vi "Interpolate Tach Pulses.vi"(5 "reset? (True)":bool=TRUE, 6 "avg on n pulses (1:no average)":i32=1, 8 "error in (no error)":errorcluster, 9 "pulse/revolution wanted":dbl=4.0 format="%.2f", 10 "pulse/revolution (1)":dbl=1.0 format="%.2f", 11 "pulse positions [s]":dbl[](array[numeric]) format="%.2f") -> (0 "error out":errorcluster, 2 "new pulse/revolution":dbl=1.0 format="%.2f", 3 "interpolated pulse positions[s]":dbl[](array[numeric]) format="%.2f")   [LabVIEW 2017, in "SoundVib_Resampling.lvlib"]
doc: "Interpolates the tachometer pulses contained in <B>pulse positions [s]</B> using <B>pulse/revolution wanted</B>. Use this VI to obtain the resample time indexes before performing resampling."
uses:
  <vilib>/addons/Sound and Vibration/Order Analysis/Resample Order Tracking/SoundVib_Resampling.lvlib
  <vilib>/addons/Sound and Vibration/Order Analysis/Tach Process/SoundVib_TachProcess.lvlib
panel:
  # "Interpolate Tach Pulses"
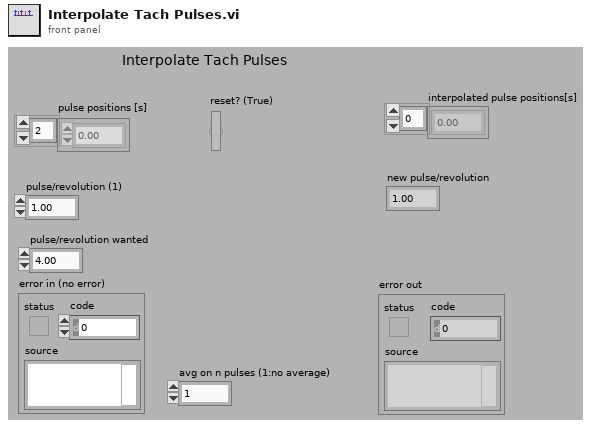
[diagram p1: front panel]
types:
  T1 = typedef "OAT Decimation Filter.ctl" = cluster{"coefficients":dbl[], "factor":i32}
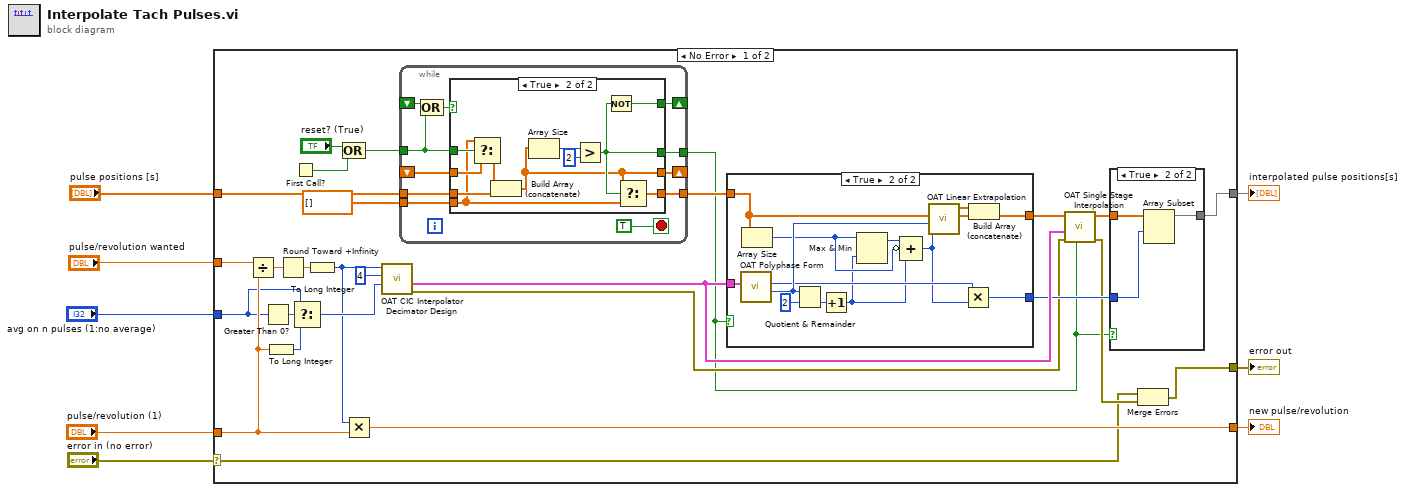
[diagram p0: block diagram]
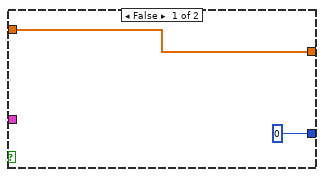
[diagram p4: hidden frame]
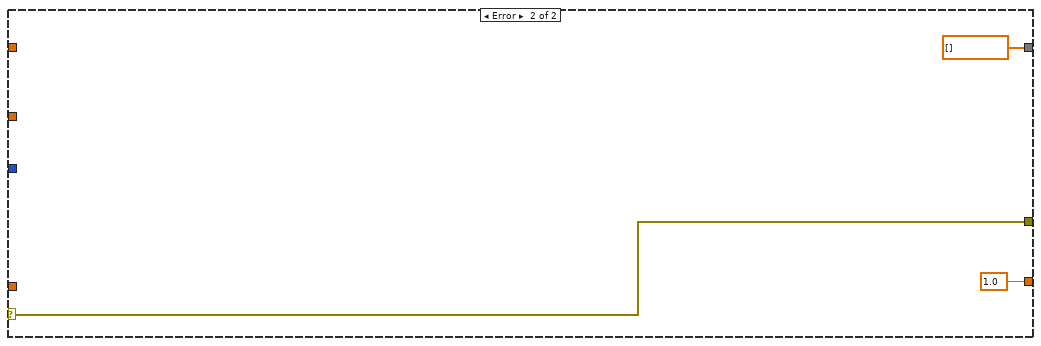
[diagram p5: hidden frame]
diagram:
  n1 = case shown="No Error" "error in (no error)" {
    selector: "error in (no error)" -> [w14 w82]
    tunnel: [w28 1.0] -> w8
    tunnel: "pulse positions [s]" -> [w13 _]
    tunnel: "pulse/revolution wanted" -> [w27 _]
    tunnel: [w26 dbl[] [] ("Y")] -> w5
    tunnel: "pulse/revolution (1)" -> [w23 _]
    tunnel: "avg on n pulses (1:no average)" -> [w21 _]
    tunnel: [w15 w82] -> w2
    frame No Error {
      n2 = Divide(x=w27, y=w23) -> (x/y=w35:dbl)
      n3 = Greater Than 0?(x=w21) -> (x > 0?=w24:bool)
      n4 = To Long Integer(number=w23) -> (32bit integer=w22:i32)
      n5 = Round Toward +Infinity(x=w35) -> (ceil(x): smallest int >= x=w34:dbl)
      n6 = First Call?() -> (First Call?: T/F=w33:bool)
      n7 = Select(t=w21, s=w24, f=w22) -> (s? t:f=w19:i32)
      n8 = To Long Integer(number=w34) -> (32bit integer=w18:i32)
      n9 = Compound Arithmetic op=OR("reset? (True)", w33) -> (w11:bool)
      n10 = Multiply(x=w18, y=w23) -> (x*y=w28:dbl)
      n11 = call <vilib>:"OAT CIC Interpolator Decimator Design.vi"("lag"=w19, "stages"=4 ("points"), "interpolation/decimation factor"=w18) -> ("error out"=w17:errorcluster, "filter"=w31:T1)  [unwired: 7 in]
      n12 = while {
        tunnel: w13 -> [w46]
        shift-right: [w41] -> _
        shift-left: _ -> [w45]
        shift-right: [w42] -> _
        shift-left: _ -> [w43]
        tunnel: w11 -> [w36]
        tunnel: dbl[] [] ("appended array") -> [w44]
        tunnel: [w40] -> w10
        tunnel: [w39] -> w9
        stop <- TRUE stop-if-true
        n13 = Compound Arithmetic op=OR(w43, w36) -> (w37:bool)
        n14 = case shown="True" w37 {
          selector: w37 -> [w47 _]
          tunnel: w46 -> [w48 w60]
          tunnel: w45 -> [_ w59]
          tunnel: w36 -> [_ w58]
          tunnel: w44 -> [w49 w50]
          tunnel: [w47 w54] -> w42
          tunnel: [w49 w51] -> w41
          tunnel: [w48 w53] -> w40
          tunnel: [_ w52] -> w39
          frame False {
          }
          frame True {
            n15 = Select(t=w50, s=w58, f=w59) -> (s? t:f=w57:dbl[])
            n16 = Build Array (concatenate)(w57, w60) -> (w51:dbl[])
            n17 = Array Size(array=w51) -> (size(s)=w56:i32)
            n18 = Greater?(x=w56, y=2) -> (0:w52:bool)
            n19 = Not(x=w52) -> (.not. x?=w54:bool)
            n20 = Select(t=w51, s=w52, f=w50) -> (s? t:f=w53:dbl[])
          }
        }
      }
      n21 = case shown="True" w9 {
        tunnel: w10 -> [w66 w72]
        tunnel: [w66 w76] -> w32
        tunnel: w31 -> [_ w79]
        tunnel: [0 w75] -> w29
        frame False {
        }
        frame True {
          n22 = call <vilib>:"OAT Polyphase Form.vi"("filter"=w79) -> ("sub filter len"=w78:i32, "decimate factor"=w69:i32)  [unwired: 8 in, 1 out]
          n23 = Array Size(array=w72) -> (size(s)=w70:i32)
          n24 = Quotient & Remainder(x=w78, y=2) -> (floor(x/y)=w74:i32)  [unwired: 1 out]
          n25 = Increment(x=w74) -> (x+1=w68:i32)
          n26 = Max & Min(x=w70, y=w68) -> (max(x,y)=w71:i32)  [unwired: 1 out]
          n27 = Compound Arithmetic op=ADD(w71, invert w70, w68) -> (w67:i32)
          n28 = call <vilib>:"OAT Linear Extrapolation.vi"("extrapolation length"=w67, "modal length"=w78, "X[n]"=w72) -> ("X[n] out"=w77:dbl[], "initail"=w73:dbl[])  [unwired: 6 in, 1 out]
          n29 = Multiply(x=w69, y=w67) -> (x*y=w75:i32)
          n30 = Build Array (concatenate)(w73, w77) -> (w76:dbl[])
        }
      }
      n31 = call <vilib>:"OAT Single Stage Interpolation.vi"("reset? (True)"=w9, "error in (no error)"=w17, "filter"=w31, "X"=w32) -> ("error out"=w16:errorcluster, "Y"=w30:dbl[])  [unwired: 6 in]
      n32 = case shown="True" w9 {
        tunnel: w30 -> [w61 w64]
        tunnel: w29 -> [_ w63]
        tunnel: [w61 w62] -> w26
        frame False {
        }
        frame True {
          n33 = Array Subset(array=w64, index=w63) -> (w62:dbl[])  [unwired: 1 in]
        }
      }
      n34 = Merge Errors(w14, w16) -> (w15:errorcluster)
    }
    frame Error {
    }
  }
  "interpolated pulse positions[s]" <- w5
  "new pulse/revolution" <- w8
  "error out" <- w2
